vi "Split Sequences.vi"(8 "error in (no error)":errorcluster, 11 "Sequence of SBlocks in":refnum<class "Sequence of SBlocks.lvclass">) -> (0 "error out":errorcluster, 1 "Kasli Order":string[](array[string]), 2 "Array of Sequences":refnum<class "Sequence of SBlocks.lvclass">[](array[class]), 3 "Sequence of SBlocks out":refnum<class "Sequence of SBlocks.lvclass">)   [LabVIEW 2020, in "Run Utilities.lvlib" / "Sequence of SBlocks.lvclass"]
uses:
  Sequence of SBlocks.lvclass
  Sequence of SBlocks.lvclass/Sequence of SBlocks.ctl
  Schedule Block/Schedule Block.lvclass
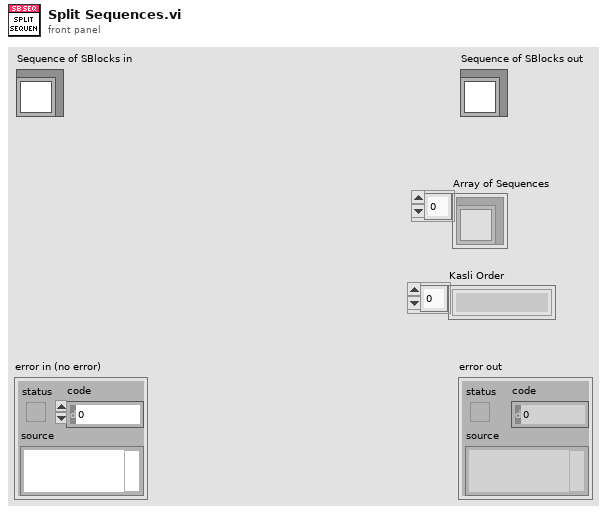
[diagram p1: front panel]
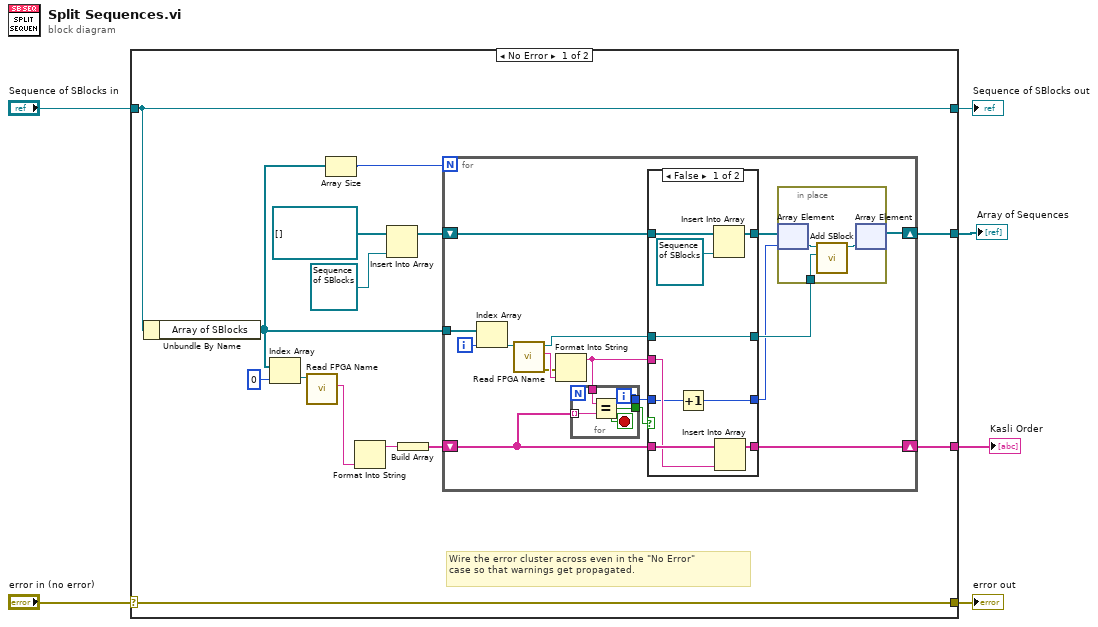
[diagram p0: block diagram]
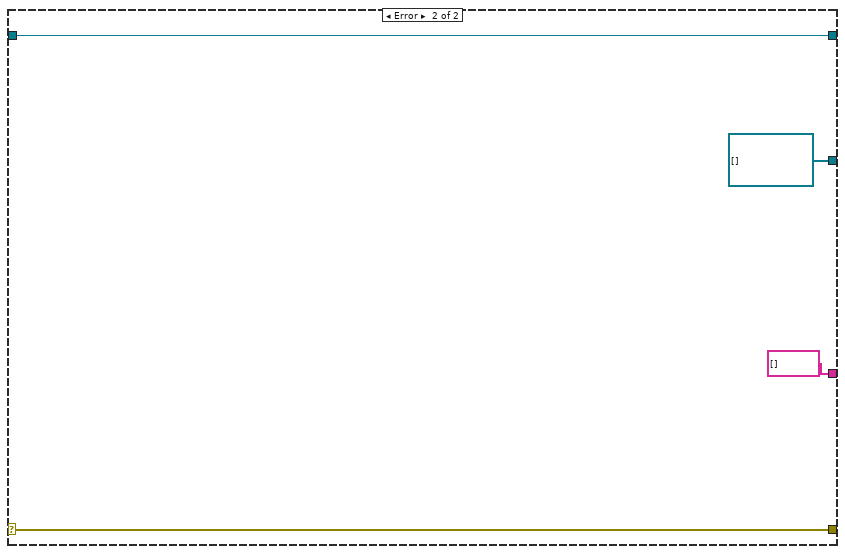
[diagram p3: hidden frame]
diagram:
  n1 = case shown="No Error" "error in (no error)" {
    selector: "error in (no error)" -> [w20 w60]
    tunnel: [w20 w60] -> w5
    tunnel: [w19 w59] -> w3
    tunnel: "Sequence of SBlocks in" -> [w19 w59]
    tunnel: [w14 refnum<class "Sequence of SBlocks.lvclass">[] []] -> w2
    tunnel: [w13 string[] []] -> w1
    frame No Error {
      # "Wire the error cluster across even in the \"No Error\"\ncase so that warnings get propagated."
      n2 = Unbundle By Name(w19) -> ("Array of SBlocks"=w17:refnum<class "Schedule Block.lvclass">[])
      n3 = Index Array(array=w17, index=0) -> (element=w7:refnum<class "Schedule Block.lvclass">)
      n4 = call-dynamic "Read FPGA Name.vi"("Schedule Block in"=w7) -> ("FPGA Name"=w8:string)  [unwired: 8 in, 2 out]
      n5 = Array Size(array=w17) -> (size(s)=w12:i32)
      n6 = Format Into String(w8) -> (resulting string=w16:string)  [unwired: 3 in, 1 out]
      n7 = Insert Into Array(array=refnum<class "Sequence of SBlocks.lvclass">[] [], new element=refnum<class "Sequence of SBlocks.lvclass"> refnum ("new element/subarray")) -> (w9:refnum<class "Sequence of SBlocks.lvclass">[])  [unwired: 1 in]
      n8 = Build Array(w16) -> (w15:string[])
      n9 = for {
        N: w12 -> [_]
        tunnel: w17 -> [w36]
        shift-right: [w35] -> w14
        shift-left: w9 -> [w33]
        shift-right: [w34] -> w13
        shift-left: w15 -> [w28]
        i -> [w30]
        n10 = Index Array(array=w36, index=w30) -> (element=w24:refnum<class "Schedule Block.lvclass">)
        n11 = call-dynamic "Read FPGA Name.vi"("Schedule Block in"=w24) -> ("error out"=w21:errorcluster, "FPGA Name"=w22:string, "Schedule Block out"=w23:refnum<class "Schedule Block.lvclass">)  [unwired: 8 in]
        n12 = Format Into String(error in=w21, w22) -> (resulting string=w27:string)  [unwired: 2 in, 1 out]
        n13 = for {
          tunnel: w28 -> [w38] mode=indexing
          tunnel: w27 -> [w40]
          tunnel: [w39] -> w29
          tunnel: [w37] -> w26
          i -> [w37]
          stop <- w39 stop-if-true
          n14 = Equal?(x=w40, y=w38) -> (x = y?=w39:bool)
        }
        n15 = case shown="False" w29 {
          tunnel: [w52 w54] -> w34
          tunnel: w33 -> [w51 w56]
          tunnel: [w50 w56] -> w32
          tunnel: [w48 w55] -> w31
          tunnel: w23 -> [w48 w55]
          tunnel: w28 -> [w47 w54]
          tunnel: w27 -> [w46 _]
          tunnel: [w44 w53] -> w25
          tunnel: w26 -> [w45 w53]
          frame False {
            n16 = Increment(x=w45) -> (x+1=w44:i32)
            n17 = Insert Into Array(array=w51, new element=refnum<class "Sequence of SBlocks.lvclass"> refnum ("new element/subarray")) -> (w50:refnum<class "Sequence of SBlocks.lvclass">[])  [unwired: 1 in]
            n18 = Insert Into Array(array=w47, new element=w46) -> (w52:string[])  [unwired: 1 in]
          }
          frame True {
          }
        }
        n19 = in-place {
          in-place-border: w31 -> [w41]
          n20 = in-place-array #1(w32, w25) -> (w43:refnum<class "Sequence of SBlocks.lvclass">)
          n21 = call-dynamic "Add SBlock.vi"("new SBlock"=w41, "Sequence of SBlocks in"=w43) -> ("Sequence of SBlocks out"=w42:refnum<class "Sequence of SBlocks.lvclass">)  [unwired: 8 in, 1 out]
          n22 = in-place-array #1(w42) -> (w35:refnum<class "Sequence of SBlocks.lvclass">[])  [unwired: 1 out]
        }
      }
    }
    frame Error {
    }
  }
  "error out" <- w5
  "Sequence of SBlocks out" <- w3
  "Array of Sequences" <- w2
  "Kasli Order" <- w1
